vi "GUI Interlock Tester-harness.vi"(11 "test case ID":string) -> (3 "result":bool)   [LabVIEW 2018]
doc: "The harness VI is executed for every test case. InstaCoverage passes the test case ID before the execution of the test case in the <b>test case ID</b> input and reads the <b>result</b> output after the execution. If the result is TRUE and no error happens during the execution, then the test case is evaluated as PASSED. If the result is false and no error happens during the execution, then the test case is evaluated as FAILED. Otherwise the test case is evaluated as ERROR.\n\nThe result of the test suite will be PASSED (FAILED) if all (at least one) test cases are PASSED (FAILED). If at least one test case in the test suite has the ERROR result, then the test suite will have ERROR result.\n\n<b>Note: </b>Don't change the connector pane of this VI.\n\nSee the Help Document for more information. (<b>Help</b> > <b>IncQuery Labs</b> > <b>InstaCoverage</b> > <b>InstaCoverage Help...</b>)"
uses:
  Libraries/Device Under Test_Cloneable_DQMH/Device Under Test_Cloneable_DQMH.lvlib
panel:
  in  "selfTestButton":bool
  in  "powerOffButton":bool
  in  "powerOnButton":bool
  # "These buttons are not inputs, they are only intended to be\n passed as reference inside this VI, for testing purposes."
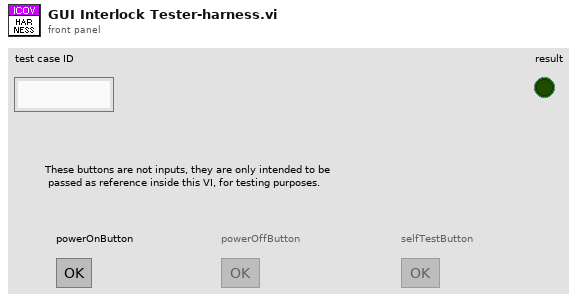
[diagram p1: front panel]
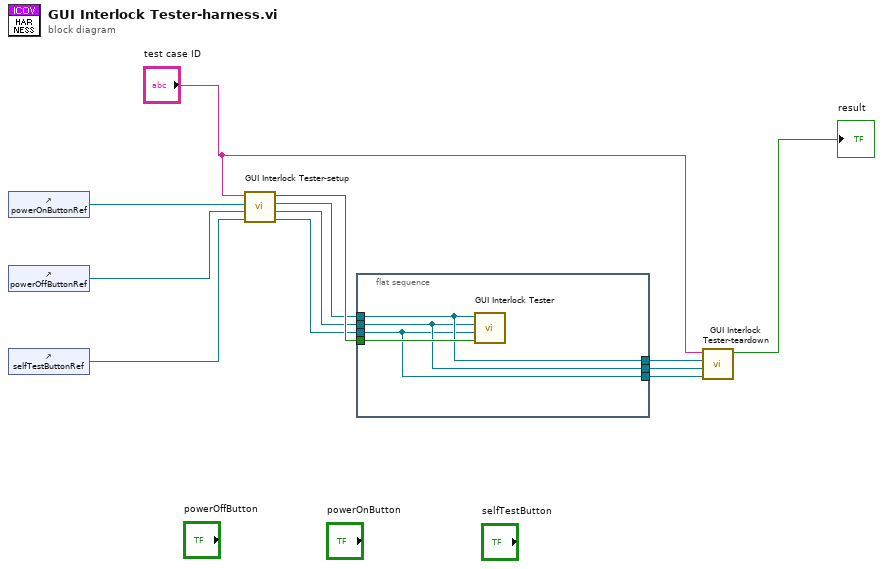
[diagram p0: block diagram]
diagram:
  n1 = control-ref of="powerOnButtonRef"() -> (w11:refnum<vi>)
  n2 = control-ref of="powerOffButtonRef"() -> (w10:refnum<vi>)
  n3 = control-ref of="selfTestButtonRef"() -> (w9:refnum<vi>)
  n4 = call "GUI Interlock Tester-setup.vi"("Self Test Button"=w9, "Power Off Button"=w10, "Power On Button"=w11, "test case ID"="test case ID") -> ("Self Test Button out"=w1:refnum<vi>, "Power Off Button out"=w2:refnum<vi>, "Power On Button out"=w3:refnum<vi>, "Power State"=w8:bool)  [unwired: 4 in]
  n5 = flat-sequence {
    tunnel: w3 -> [w15]
    tunnel: w2 -> [w14]
    tunnel: w1 -> [w13]
    tunnel: w8 -> [w16]
    tunnel: [w15] -> w6
    tunnel: [w14] -> w5
    tunnel: [w13] -> w4
    frame #0 {
      n6 = call "GUI Interlock Tester.vi"("Power State"=w16, "Self Test Button"=w13, "Power Off Button"=w14, "Power On Button"=w15) -> ()  [unwired: 8 in]
    }
  }
  n7 = call "GUI Interlock Tester-teardown.vi"("Self Test Button"=w4, "Power Off Button"=w5, "Power On Button"=w6, "test case ID"="test case ID") -> ("result"=→"result":bool)  [unwired: 7 in]
